vi "HumanSwerveDrive.vi"(9 "Rotation":dbl, 10 "Y":dbl, 11 "X":dbl) -> (1 "A":dbl, 2 "Y":dbl, 3 "X":dbl)   [LabVIEW 2020]
uses:
  <vilib>/Rock Robotics/WPI/ThirdParty/JAS_Junk/TrajLib/Trajectory_Library.lvlib
panel:
  # "we switched these, hopefully it is right"
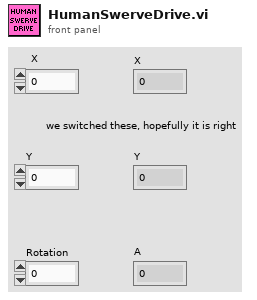
[diagram p1: front panel]
types:
  T1 = typedef "Trajectory_Library.lvlib/ROTATION2D.ctl" = cluster{"VALUE":dbl, "COS":dbl, "SIN":dbl}
  T2 = typedef "Trajectory_Library.lvlib/TRANSLATION2D.ctl" = cluster{"X":dbl, "Y":dbl}
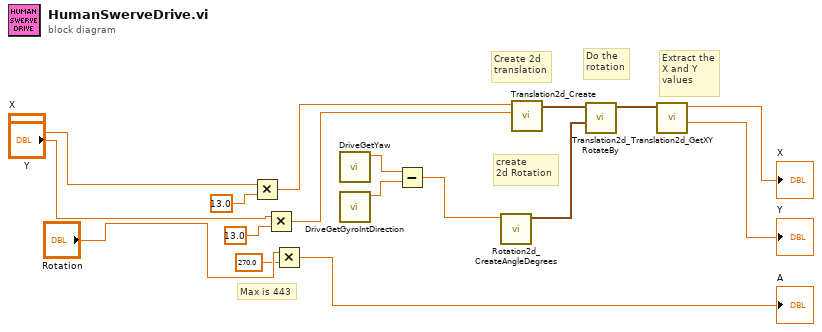
[diagram p0: block diagram]
diagram:
  # "Extract the\nX and Y \nvalues"
  # "Do the \nrotation"
  # "Create 2d\ntranslation"
  # "create\n2d Rotation"
  # "Max is 443"
  n1 = Multiply(x="X", y=13.0) -> (x*y=w8:dbl)
  n2 = Multiply(x="Y", y=13.0) -> (x*y=w9:dbl)
  n3 = Multiply(x="Rotation", y=270.0) -> (x*y=→"A":dbl)
  n4 = call "DriveGetYaw.vi"() -> ("Yaw"=w15:dbl)  [unwired: 11 in]
  n5 = call "DriveGetGyroIntDirection.vi"() -> ("GyroIntDirection"=w16:dbl)  [unwired: 11 in]
  n6 = Subtract(x=w15, y=w16) -> (x-y=w17:dbl)
  n7 = call <vilib>:"Rotation2d_CreateAngleDegrees.vi"("Angle_Degrees"=w17) -> ("ROTATION"=w11:T1)  [unwired: 10 in]
  n8 = call <vilib>:"Translation2d_Create.vi"("Y"=w9, "X"=w8) -> ("TRANSLATION"=w10:T2)  [unwired: 9 in]
  n9 = call <vilib>:"Translation2d_RotateBy.vi"("other Rotation"=w11, "In Translation"=w10) -> ("Out Translation"=w12:T2)  [unwired: 9 in]
  n10 = call <vilib>:"Translation2d_GetXY.vi"("In Translation"=w12) -> ("Y"=→"Y":dbl, "X"=→"X":dbl)  [unwired: 9 in]
